vi "GetParamTxtPath.vi"(2 "Checksums in":string[](array[string]), 3 "System":u16(ring) items=["Cusp", "Positron", "Musashi"], 4 "Action index path":path=path "C:/CuspControl/GPIB and Network/ActionIndex.txt") -> (0 "Checksums out":string[](array[string])=["c81e728d9d4c2f636f067f89cc14862c", "9d7a1433adf69f3943457e7b4a446b32", "cfcd208495d565ef66e7dff9f98764da", "93a1f446527426f1d8a59809b8859b3c", "3a0566edaf92ce782fb91852dfd8d01e", "3ee8446ffde602473630d63e302587c0", "4256d504e6b8c2781ea4473923f403d7", "86bcf6b5ddbd761c8ce10b0764dd2628", "0e44fccf2678f95aa60d612e6c175696", "94179c42c6d4654145c0effe2597ac22", "e526fc795b8cf78588dc4cfc32651329", "09447ed7f93f5dd16b71de533d59bf94", "2325305ce2dedaff3f1e20b84478eaf0", "cfcd208495d565ef66e7dff9f98764da", "e45842c4ceef846afee3ec17e4b810cb", "184713af2d87a1800f144b4109514265"], 1 "Paths out":path[](array[path])=[path "C:/CuspControl/GPIB and Network/Cusp/HVpulser.txt"])   [LabVIEW 2018]
panel:
  # "LEAVE \"CHECKSUMS IN\" DEFAULT VALUE = NULL (EMPTY)\notherwise the conditional won't work when this VI is used to initialize"
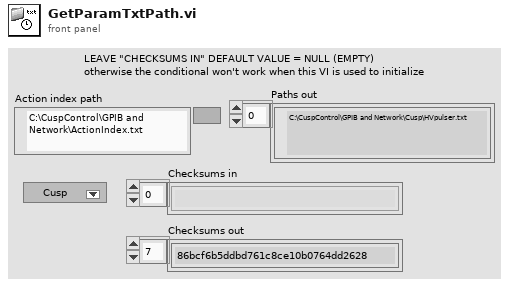
[diagram p1: front panel]
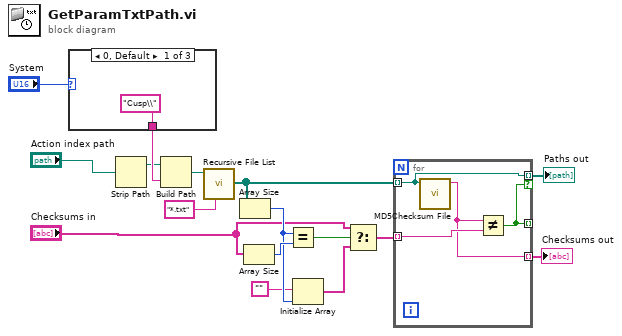
[diagram p0: block diagram]
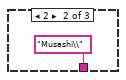
[diagram p2: hidden frame]
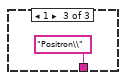
[diagram p3: hidden frame]
diagram:
  n1 = case shown="0, Default" "System" {
    tunnel: ["Cusp\\" ("name or relative path") "Musashi\\" ("name or relative path") "Positron\\" ("name or relative path")] -> w13
    frame 0, Default {
    }
    frame 2 {
    }
    frame 1 {
    }
  }
  n2 = Strip Path(path="Action index path") -> (stripped path=w12:path)  [unwired: 1 out]
  n3 = Build Path(base path=w12, name or relative path=w13) -> (appended path=w14:path)
  n4 = call <vilib>:"Recursive File List.vi"("pattern"="*.txt", "Folder Path"=w14) -> ("All Files in Dir"=w8:path[])  [unwired: 5 in, 4 out]
  n5 = Array Size(array=w8) -> (size(s)=w5:i32)
  n6 = Array Size(array="Checksums in") -> (size(s)=w7:i32)
  n7 = Equal?(x=w5, y=w7) -> (x = y?=w6:bool)
  n8 = Initialize Array("", w5) -> (w2:string[])
  n9 = Select(t="Checksums in", s=w6, f=w2) -> (s? t:f=w9:string[])
  n10 = for {
    tunnel: w8 -> [w22] mode=indexing
    tunnel: w9 -> [w23] mode=indexing
    tunnel: [w22] -> w16 mode=indexing if=w20
    tunnel: [w21] -> w4 mode=indexing
    tunnel: [w20] -> _ mode=indexing
    n11 = call <vilib>:"MD5Checksum File.vi"("Path"=w22) -> ("MD5 message-digest"=w21:string)  [unwired: 9 in, 1 out]
    n12 = Not Equal?(x=w21, y=w23) -> (x != y?=w20:bool)
  }
  "Paths out" <- w16
  "Checksums out" <- w4
